vi "Create JSON Schema.vi"() -> ()   [LabVIEW 2023, in "JSON Schema Generator.lvlib"]
uses:
  JSON Schema Generator.lvlib
  7dc4fba5-8a80-492e-b267-0080a53f7d5c.vi
  <vilib>/JDP Science/JSONtext/Variant to JSON Text.vi
  <vilib>/JDP Science/JSONtext/LVClass Serializer/JSONtext LVClass Serializer.lvclass
  <vilib>/JDP Science/JSONtext/JSONtext.lvlib
panel:
  out "error out 2":errorcluster
  out "<JSON>":string
  out "error out":errorcluster
  in  "Example Cluster":T1={"ProductId"=1, "productName"="A green door", "price"=12.5, "tags"=["home", "green"], "ProductNumber"=1, "ProductInfoInternal"={"ProductState"=enum."Active", "State Info"={"Date"="", "Time"=0.0}}, "Product History"=[]}
  out "Invalid":bool
  in  "error in (no error)":errorcluster
  in  "Description":string
  in  "Title":string="test"
  out "JSON Schema out":string caption="JSON Schema"
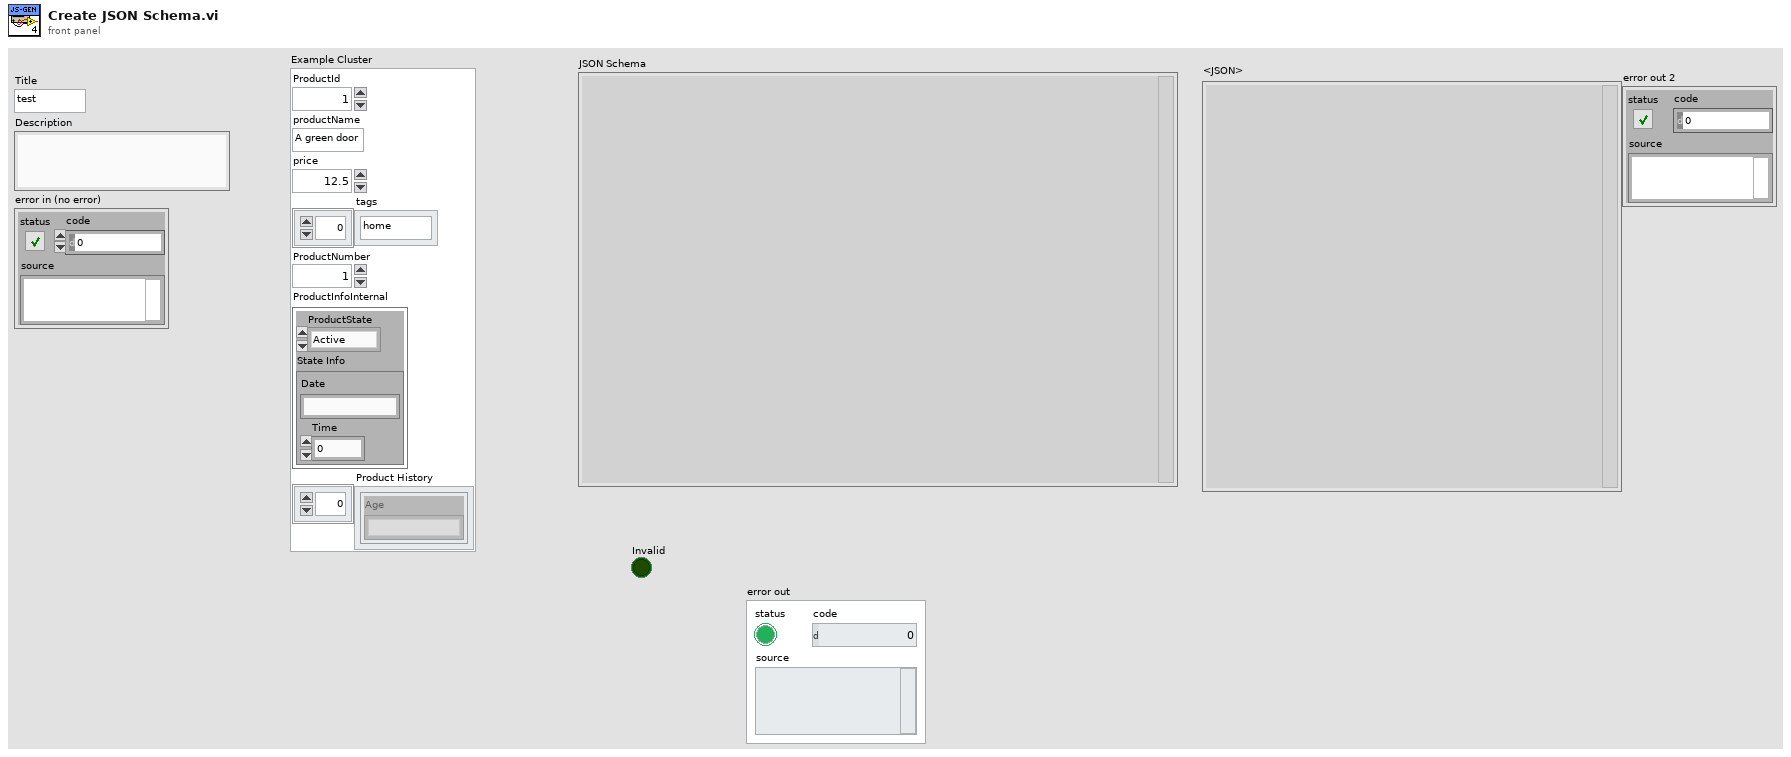
[diagram p1: front panel]
types:
  T1 = cluster{"ProductId":i32, "productName":string, "price":dbl, "tags":string[], "ProductNumber":i32, "ProductInfoInternal":cluster{"ProductState":enum16{"Active", "InActive"}, "State Info":cluster{"Date":string, "Time":dbl}}, "Product History":cluster{"Age":string}[]}
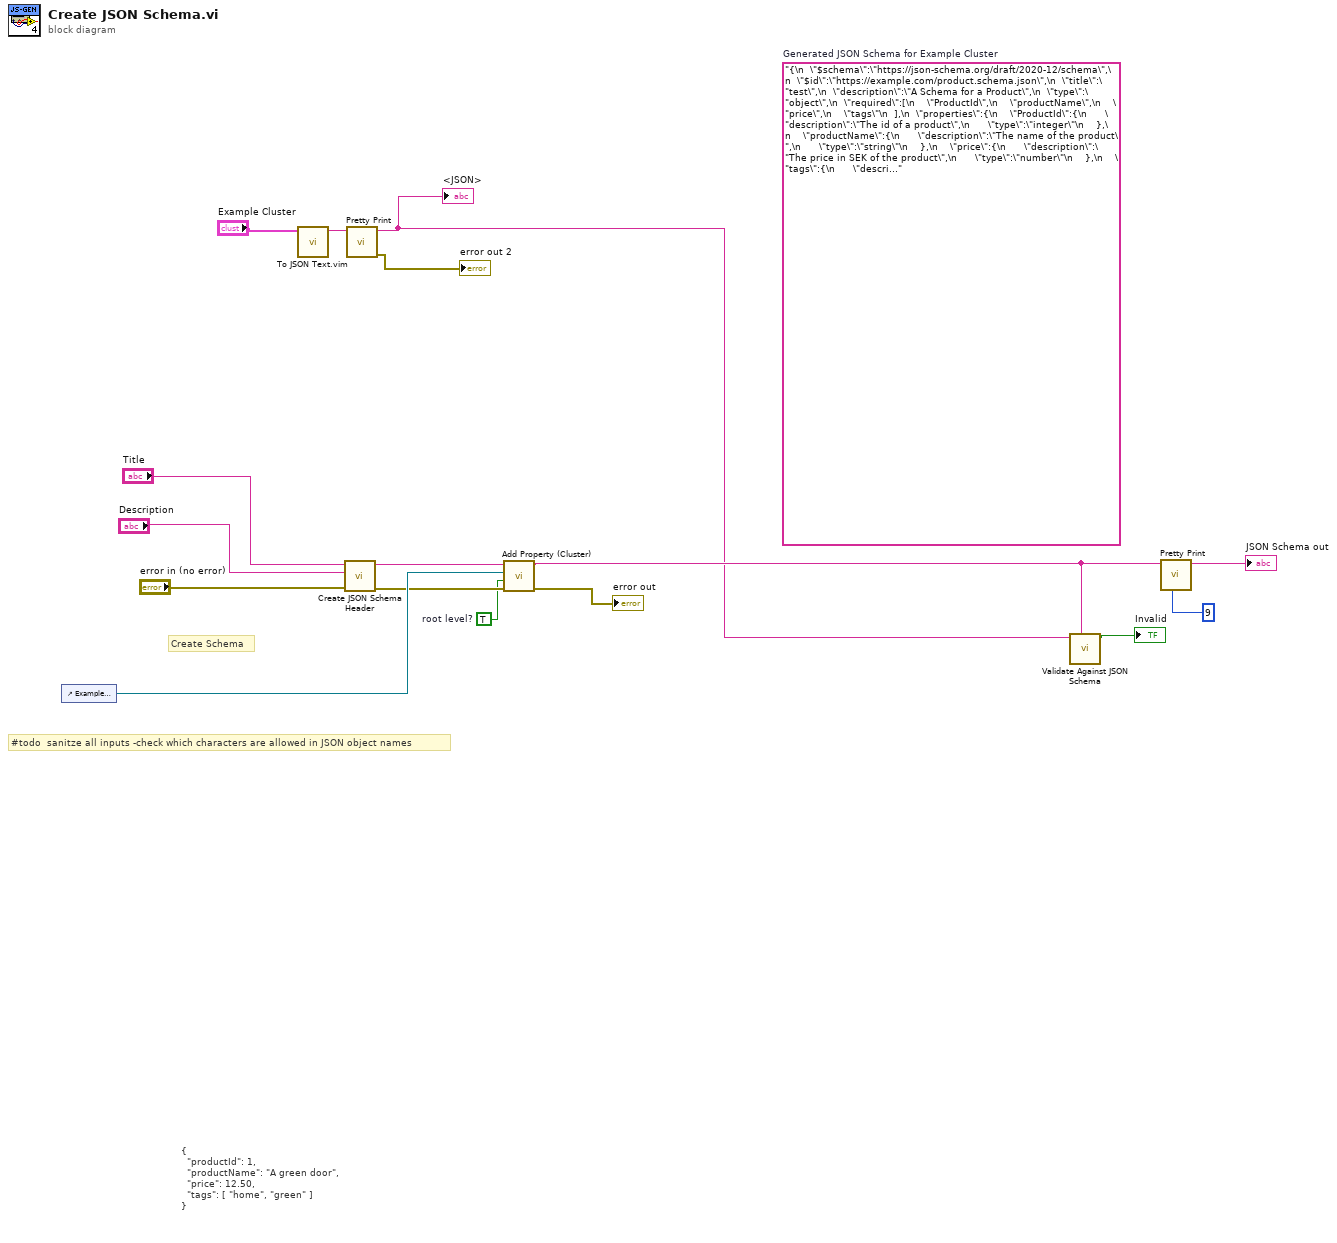
[diagram p0: block diagram]
diagram:
  w1 = TRUE  # root level?
  (unwired) "{\n  \"$schema\":\"https://json-schema.org/draft/2020-12/schema\",\n  \"$id\":\"https://example.com/product.schema.json\",\n  \"title\":\"test\",\n  \"description\":\"A Schema for a Product\",\n  \"type\":\"object\",\n  \"required\":[\n    \"ProductId\",\n    \"productName\",\n    \"price\",\n    \"tags\"\n  ],\n  \"properties\":{\n    \"ProductId\":{\n      \"description\":\"The id of a product\",\n      \"type\":\"integer\"\n    },\n    \"productName\":{\n      \"description\":\"The name of the product\",\n      \"type\":\"string\"\n    },\n    \"price\":{\n      \"description\":\"The price in SEK of the product\",\n      \"type\":\"number\"\n    },\n    \"tags\":{\n      \"description\":\"Tags accociated with the product\",\n      \"type\":\"array\",\n      \"items\":{\"type\":\"string\"}\n    }\n  }\n}"  # Generated JSON Schema for Example Cluster
  # "#todo  sanitze all inputs -check which characters are allowed in JSON object names"
  # "Create Schema"
  # "{\n  \"productId\": 1,\n  \"productName\": \"A green door\",\n  \"price\": 12.50,\n  \"tags\": [ \"home\", \"green\" ]\n}"
  n1 = control-ref of="Example Cluster"() -> (w9:refnum<vi>)
  n2 = call "To JSON Text.vim"("Anything"="Example Cluster") -> ("<JSON>"=w4:string)  [unwired: 9 in, 1 out]
  n3 = call "Create JSON Schema Header.vi"("error in (no error)"="error in (no error)", "Description"="Description", "Title"="Title") -> ("error out"=w6:errorcluster, "JSON Schema out"=w10:string)  [unwired: 7 in]
  n4 = call <vilib>:"Pretty Print.vi"("JSON"=w4) -> ("error out"=→"error out 2":errorcluster, "<JSON>"=w2:string)  [unwired: 8 in, 1 out]
  "<JSON>" <- w2
  n5 = call "Add Property (Cluster).vi"("error in (no error)"=w6, "root level?"=w1, "Cluster in"=w9, "JSON Schema in"=w10) -> ("error out"=→"error out":errorcluster, "JSON Schema out"=w7:string)  [unwired: 6 in]
  n6 = call <vilib>:"Validate Against JSON Schema.vi"("JSON Schema"=w7, "JSON"=w2) -> ("Invalid"=→"Invalid":bool)  [unwired: 5 in, 4 out]
  n7 = call <vilib>:"Pretty Print.vi"("Pretty Print Levels"=9, "JSON"=w7) -> ("<JSON>"=→"JSON Schema out":string)  [unwired: 7 in, 2 out]
